vi "Save Pressure from Web.vi"(2 "error in":errorcluster) -> (0 "error out":errorcluster, 1 "Pressure":dbl)   [LabVIEW 2016]
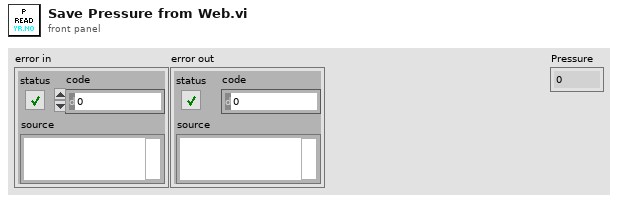
[diagram p1: front panel]
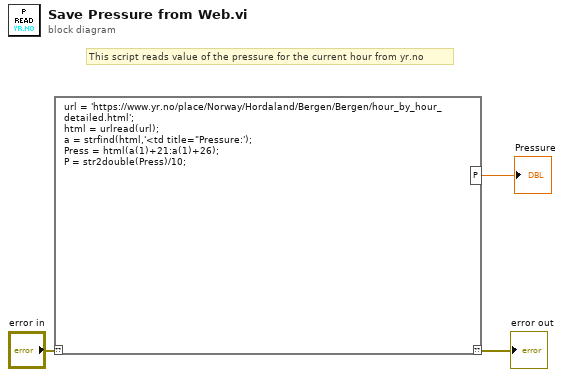
[diagram p0: block diagram]
diagram:
  # "This script reads value of the pressure for the current hour from yr.no"
  n1 = script code="url = 'https://www.yr.no/place/Norway/Hordaland/Bergen/Bergen/hour_by_hour_detailed.html';\nhtml = urlread(url);\na = strfind(html,'<td title=\"Pressure:');\nPress = html(a(1)+21:a(1)+26);\nP = str2double(Press)/10;"("??"="error in") -> ("??"=→"error out":errorcluster, "P"=→"Pressure":dbl)
